vi "CalcRateSubVI.vi"(10 "Elapsed Time (s)":dbl, 11 "Changed Quantity":dbl) -> (3 "Rate of Change":dbl)   [LabVIEW 2019]
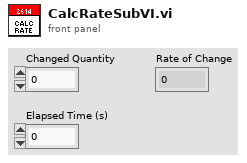
[diagram p1: front panel]
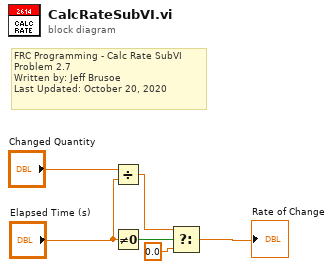
[diagram p0: block diagram]
diagram:
  # "FRC Programming - Calc Rate SubVI\nProblem 2.7\nWritten by: Jeff Brusoe\nLast Updated: October 20, 2020"
  n1 = Divide(x="Changed Quantity", y="Elapsed Time (s)") -> (x/y=w3:dbl)
  n2 = Not Equal To 0?(x="Elapsed Time (s)") -> (x != 0?=w1:bool)
  n3 = Select(t=w3, s=w1, f=0.0) -> (s? t:f=→"Rate of Change":dbl)
